vi "Demo.vi"() -> ()   [LabVIEW 2014, in "BT.lvlib" / "BT.lvclass"]
uses:
  BT.lvclass
panel:
  in  "Device Name Or Device Address":string
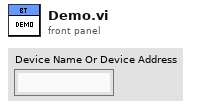
[diagram p1: front panel]
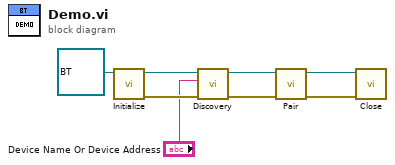
[diagram p0: block diagram]
diagram:
  n1 = call-dynamic "Initialize.vi"("BT in"=refnum<class "BT.lvclass"> refnum) -> ("error out"=w7:errorcluster, "BT out"=w8:refnum<class "BT.lvclass">)  [unwired: 9 in]
  n2 = call "Discovery.vi"("error in (no error)"=w7, "Device Name Or Device Address"="Device Name Or Device Address", "BT in"=w8) -> ("error out"=w5:errorcluster, "BT out"=w6:refnum<class "BT.lvclass">)  [unwired: 7 in]
  n3 = call "Pair.vi"("error in (no error)"=w5, "BT in"=w6) -> ("error out"=w3:errorcluster, "BT out"=w4:refnum<class "BT.lvclass">)  [unwired: 8 in]
  n4 = call "Close.vi"("error in (no error)"=w3, "BT in"=w4) -> ()  [unwired: 8 in, 2 out]
